vi "Enumerate Devices.vi"(8 "error in (no error)":errorcluster, 11 "CameraManager":refnum<data-value>) -> (0 "error out":errorcluster, 2 "Devices":map{string, T1}(c390), 3 "CameraManager (duplicate)":refnum<data-value>)   [LabVIEW 2020, in "g_ar_toolkit.capture.lvlib" / "CameraManager.lvclass"]
uses:
  CameraManager.lvclass
  Stream Enumeration.ctl
  Stream Parameters.ctl
  CameraManager.lvclass/CameraManager.ctl
  bin/g_ar_toolkit.1.32.dll
  Pixel Format.ctl
  Format.ctl
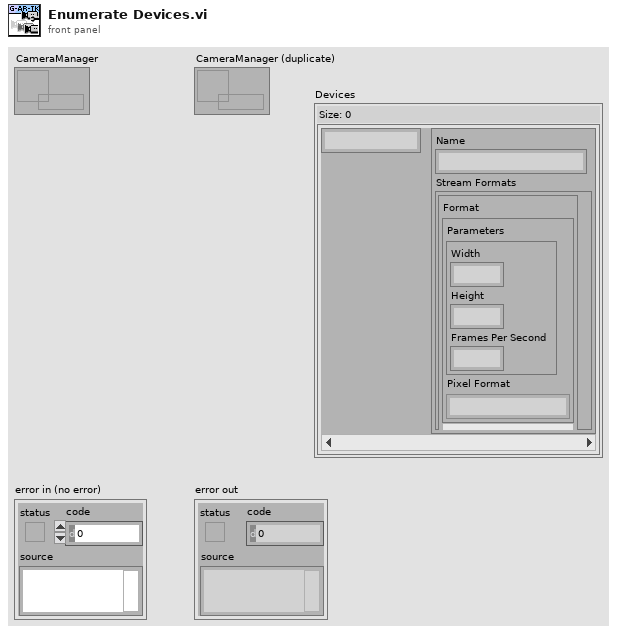
[diagram p1: front panel]
types:
  T1 = typedef "g_ar_toolkit.capture.lvlib/CameraManager.lvclass/Stream Enumeration.ctl" = cluster{"Name":string, "Stream Formats":set{T2}}
  T2 = typedef "g_ar_toolkit.capture.lvlib/CameraManager.lvclass/Format.ctl" = cluster{"Parameters":T3, "Pixel Format":T4}
  T3 = typedef "g_ar_toolkit.capture.lvlib/CameraManager.lvclass/Stream Parameters.ctl" = cluster{"Width":u16, "Height":u16, "Frames Per Second":u8}
  T4 = typedef "g_ar_toolkit.capture.lvlib/CameraManager.lvclass/Pixel Format.ctl" = enum32{"UNKNOWN", "RGB24", "RGB32", "YUV", "NV12", "MJPEG", "H264"}
  T5 = cluster{"id":string, "name":string, cluster{"pixel-format":T4, "width":u32, "height":u32, "fps_n":u32, "fps_d":u32}[]}[]
  T6 = cluster{"pixel-format":T4, "width":u32, "height":u32, "fps_n":u32, "fps_d":u32}[]
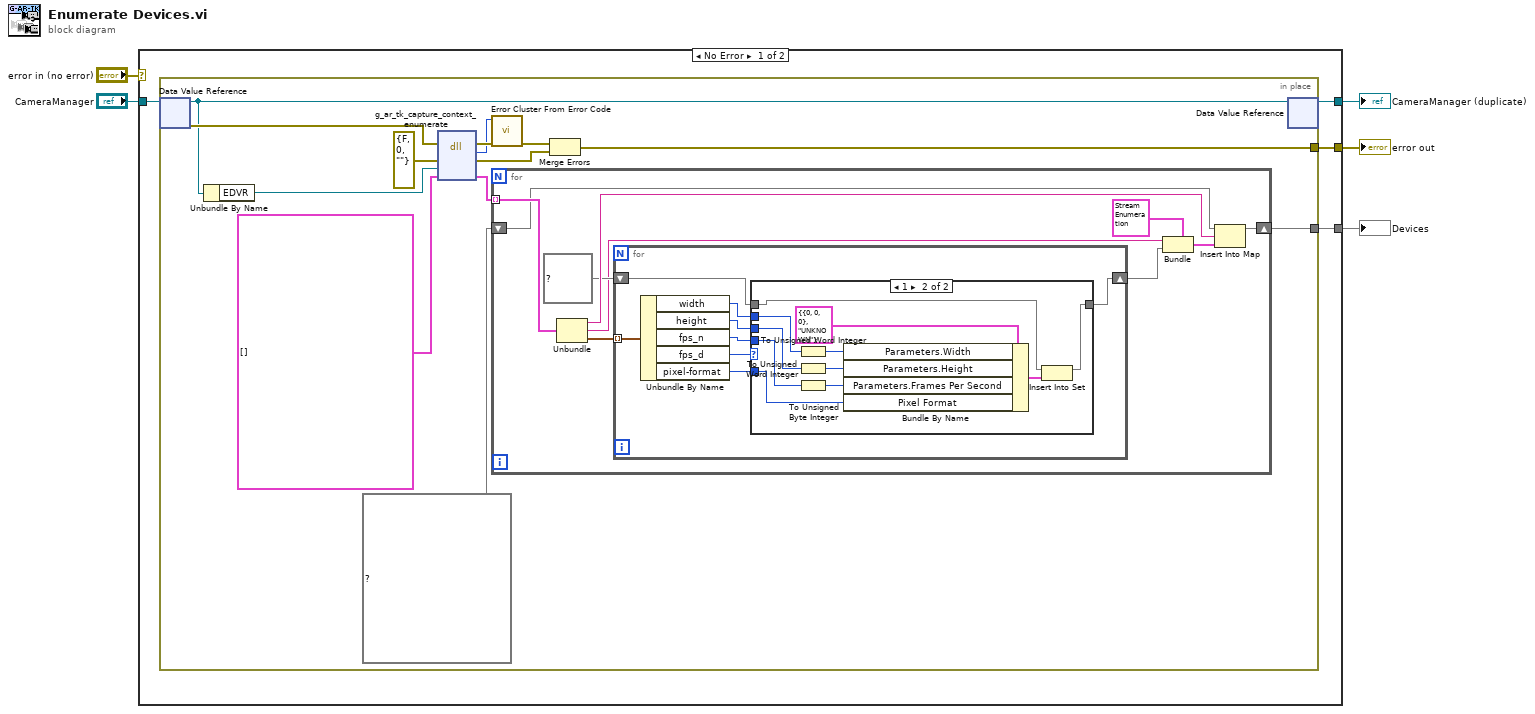
[diagram p0: block diagram]
diagram:
  n1 = case shown="No Error" "error in (no error)" {
    selector: "error in (no error)" -> [_ w54]
    tunnel: [w8 w54] -> w4
    tunnel: [w7 w53] -> w2
    tunnel: "CameraManager" -> [w9 w53]
    tunnel: [w6 _] -> w1
    frame No Error {
      n2 = in-place {
        in-place-border: [w15] -> w8
        in-place-border: [w10] -> w6
        n3 = in-place-dvr #1(w9) -> (w14:refnum<class "CameraManager.lvclass">, w16:errorcluster)
        n4 = Unbundle By Name(w14) -> ("EDVR"=w18:refnum<data-value>)
        n5 = dll-call lib="C:/serenial/libraries/g-augmented-reality-toolkit/LabVIEW/bin/g_ar_toolkit.1.*.*" fn="g_ar_tk_capture_context_enumerate"(error in=w16, "error_cluster"=errorcluster {"status"=FALSE, "code"=0, "source"=""} ("error constant"), "EDVR"=w18, "device_list"=T5 []) -> (error out=w22:errorcluster, "MgErr"=w17:i32, "error_cluster"=w19:errorcluster, "device_list"=w12:T5)  [unwired: 3 in, 1 out]
        n6 = call <vilib>:"Error Cluster From Error Code.vi"("error in (no error)"=w22, "error code (0)"=w17) -> ("error out"=w21:errorcluster)  [unwired: 7 in]
        n7 = for {
          tunnel: w12 -> [w32] mode=indexing
          shift-right: [w24] -> w10
          shift-left: map{string, T1} {} ("Size: 0") -> [w23]
          n8 = Unbundle(w32) -> ("id"=w31:string, "name"=w27:string, w30:T6)
          n9 = for {
            tunnel: w30 -> [w40] mode=indexing
            shift-right: [w36] -> w28
            shift-left: set{T2} {} ("Size: 0") -> [w35]
            n10 = Unbundle By Name(w40) -> ("width"=w37:u32, "height"=w38:u32, "fps_n"=w39:u32, "fps_d"=w33:u32, "pixel-format"=w34:T4)
            n11 = case shown="1" w33 {
              tunnel: w39 -> [_ w52]
              tunnel: w38 -> [_ w51]
              tunnel: w37 -> [_ w50]
              tunnel: [w41 w49] -> w36
              tunnel: w35 -> [w41 w48]
              tunnel: w34 -> [_ w42]
              frame Default {
              }
              frame 1 {
                n12 = To Unsigned Word Integer(number=w50) -> (unsigned 16bit integer=w46:u16)
                n13 = To Unsigned Word Integer(number=w51) -> (unsigned 16bit integer=w45:u16)
                n14 = To Unsigned Byte Integer(number=w52) -> (unsigned 8bit integer=w43:u8)
                n15 = Bundle By Name(cluster=T2 {"Parameters"={"Width"=0, "Height"=0, "Frames Per Second"=0}, "Pixel Format"=enum."UNKNOWN"} ("Format"), "Parameters.Width"=w46, "Parameters.Height"=w45, "Parameters.Frames Per Second"=w43, "Pixel Format"=w42) -> (w44:T2)
                n16 = Insert Into Set(10:w44, 11:w48) -> (3:w49:set{T2})  [unwired: 1 out]
              }
            }
          }
          n17 = Bundle(cluster=T1 {"Name"="", "Stream Formats"={}} ("Enumeration"), "Name"=w27, "Stream Formats"=w28) -> (w26:T1)
          n18 = Insert Into Map(map in=w23, key=w31, value=w26) -> (map out=w24:map{string, T1})  [unwired: 2 out]
        }
        n19 = Merge Errors(w21, w19) -> (w15:errorcluster)
        n20 = in-place-dvr #1(w14) -> (w7:refnum<data-value>)  [unwired: 1 out]
      }
    }
    frame Error {
    }
  }
  "error out" <- w4
  "CameraManager (duplicate)" <- w2
  "Devices" <- w1
